vi "FMA1600A General Setup.vi"(5 "Gas Type":T5, 6 "Baud Rate":T2(ring)=enum."19200", 7 "Unit ID":string, 8 "error in (no error)":errorcluster, 9 "Select Gas?":bool=TRUE, 10 "Set STP Register":bool, 11 "VISA Refnum in":refnum<visa-resource-name>) -> (0 "error out":errorcluster, 1 "Data Frame Format":T1, 2 "Measurement Units":T3, 3 "VISA Refnum out":refnum<visa-resource-name>)   [LabVIEW 2019]
uses:
  Type Definitions/FMA1600A Gas Type.ctl
  Type Definitions/FMA1600A Units String.ctl
  Alicat Gas Meter Driver/Sub-VIs/Units of Measure.ctl
  Alicat Gas Meter Driver/Sub-VIs/Data Frame.ctl
  Type Definitions/FMA1600A Commands.ctl
  <vilib>/Utility/error.llb/whitespace.ctl
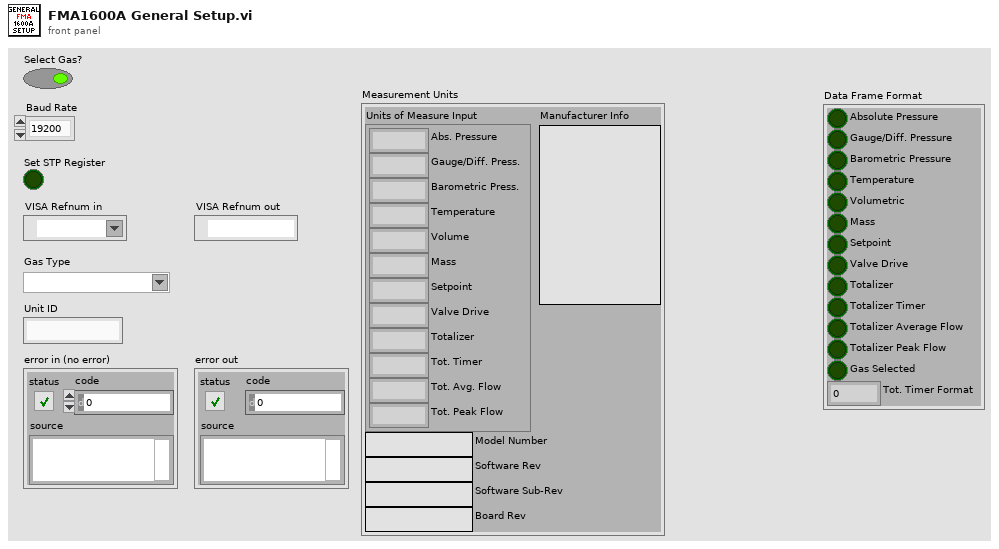
[diagram p1: front panel]
types:
  T1 = typedef "Data Frame.ctl" = cluster{"Absolute Pressure":bool, "Gauge/Diff. Pressure":bool, "Barometric Pressure":bool, "Temperature":bool, "Volumetric":bool, "Mass":bool, "Setpoint":bool, "Valve Drive":bool, "Totalizer":bool, "Totalizer Timer":bool, "Totalizer Average Flow":bool, "Totalizer Peak Flow":bool, "Gas Selected":bool, "Tot. Timer Format":u16}
  T2 = enum8{"2400", "9600", "19200", "38400", "57600", "115200", "Unknown"}
  T3 = typedef "FMA1600A Units String.ctl" = cluster{"Software Rev":string, "Model Number":string, "Manufacturer Info":string, "Software Sub-Rev":string, "Board Rev":string, "Units of Measure Input":T4}
  T4 = typedef "Units of Measure.ctl" = cluster{"Abs. Pressure":string, "Gauge/Diff. Press.":string, "Barometric Press.":string, "Temperature":string, "Volume":string, "Mass":string, "Setpoint":string, "Valve Drive":string, "Totalizer":string, "Tot. Timer":string, "Tot. Avg. Flow":string, "Tot. Peak Flow":string}
  T5 = typedef "FMA1600A Gas Type.ctl" = string
  T6 = cluster{"Valve Drive":bool, "Totalizer":bool, "Totalizer Timer":bool, "Totalizer Peak Flow":bool, "Show Abs., Gauge\nand Baro. pressures":bool}
  T7 = cluster{"Pressure(s)":bool, "Temperature":bool, "Volumetric":bool, "Mass":bool, "Totalizer Average Flow":bool, "Gas Selected":bool}
  T8 = typedef "whitespace.ctl" = u16
  T9 = typedef "FMA1600A Commands.ctl" = string
  T10 = cluster{"Unit ID":string, "Baud Rate":enum8{"2400", "9600", "19200", "38400", "57600", "115200", "Unknown"}, "VISA Sesssion In":refnum<visa-resource-name>}
  T11 = cluster{"Abs. Pressure":string, "Gauge/Diff. Press.":string, "Barometric Press.":string, "Temperature":string, "Volume":string, "Mass":string, "Setpoint":string, "Valve Drive":string, "Totalizer":string, "Tot. Timer":string, "Tot. Avg. Flow":string, "Tot. Peak Flow":string}
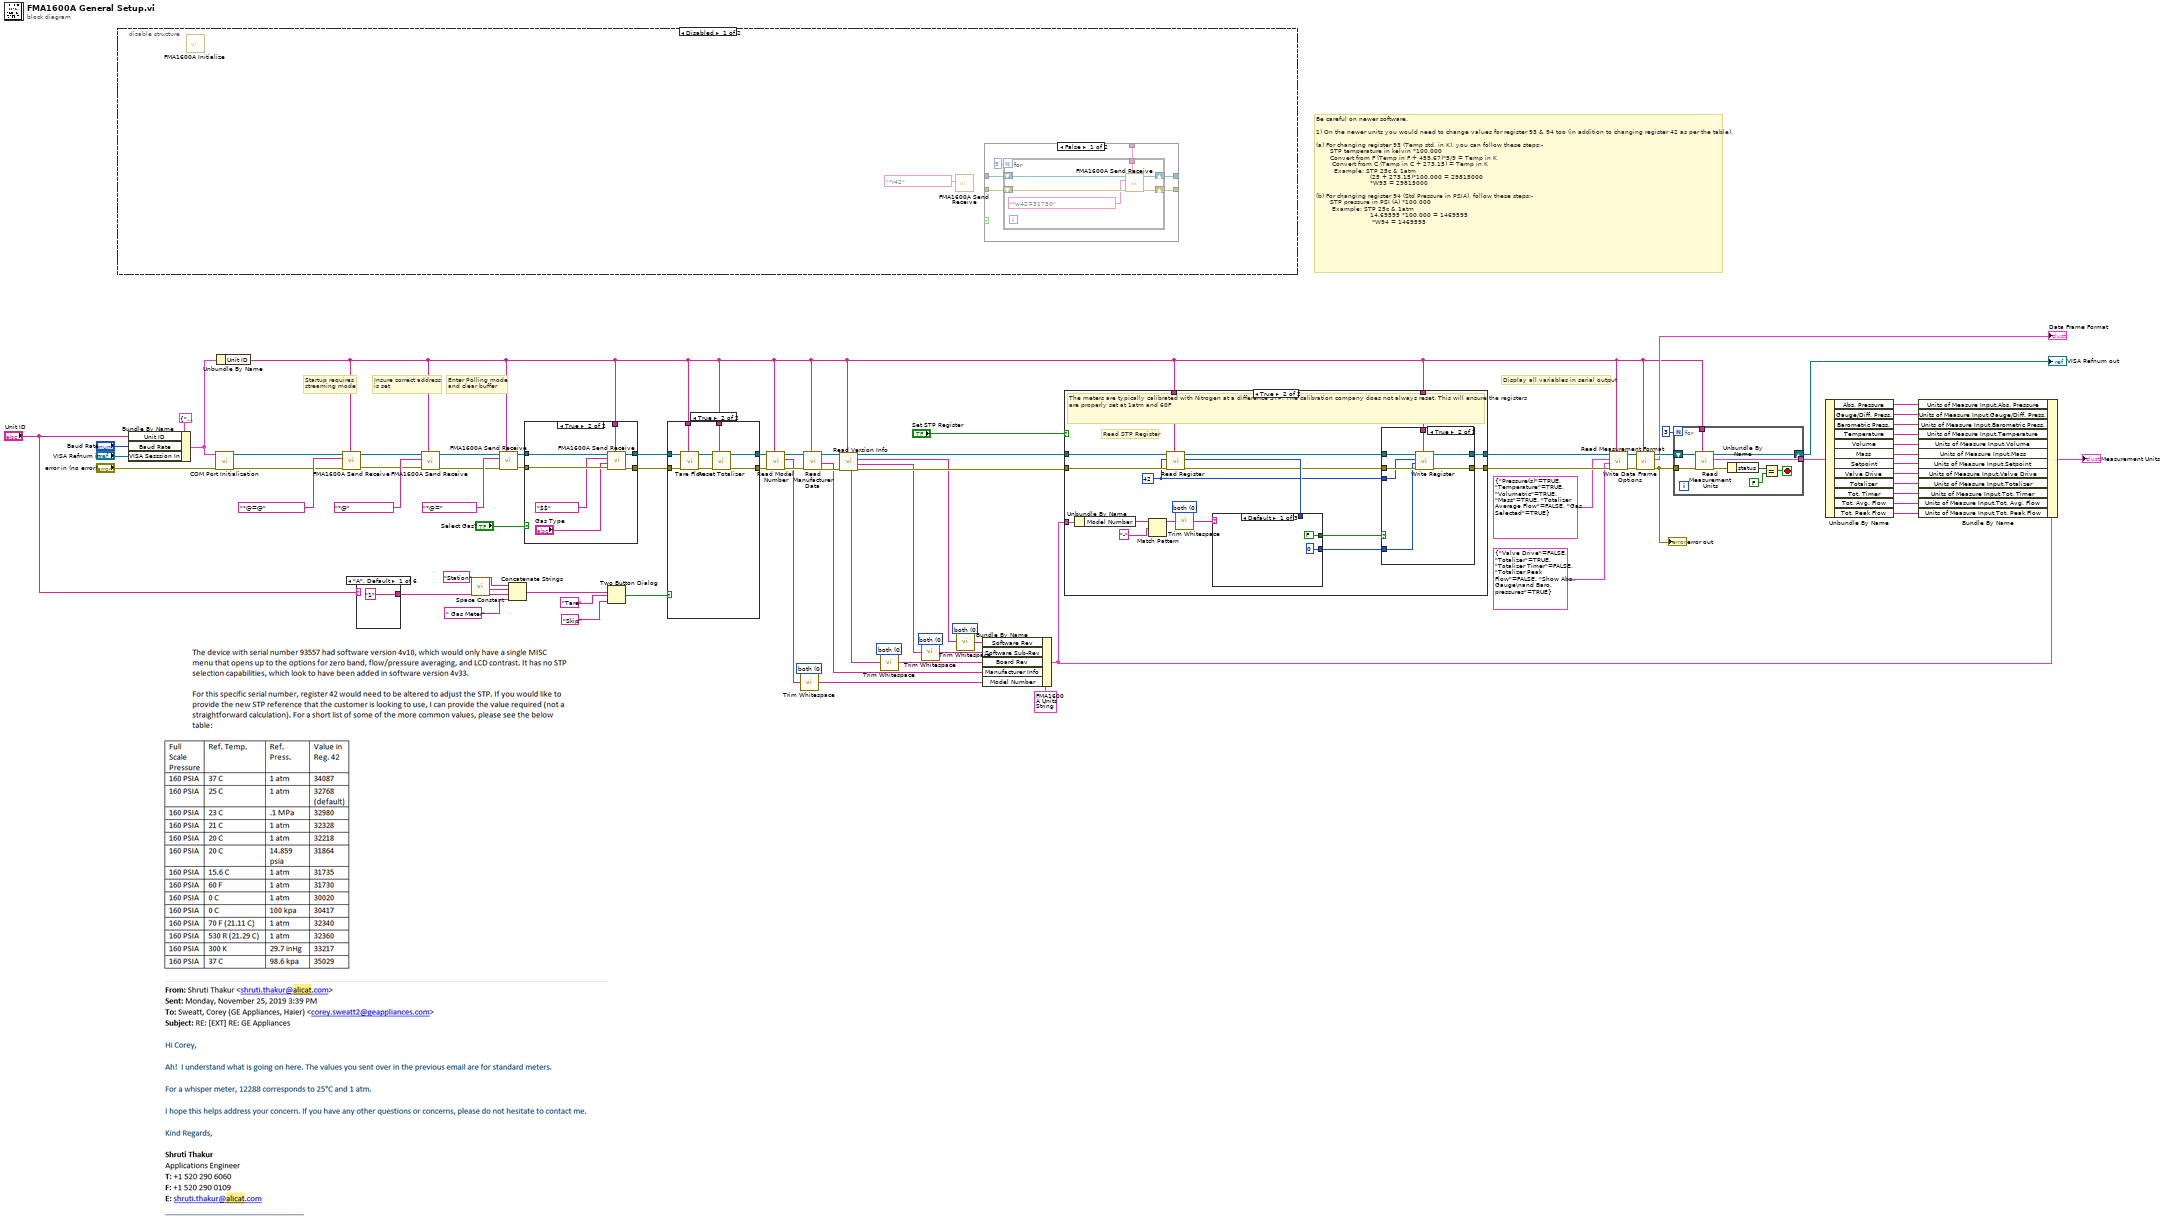
[diagram p0: block diagram]
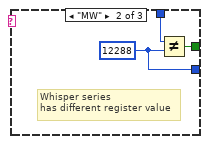
[diagram p7: hidden frame]
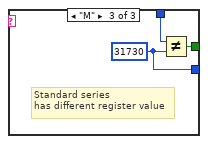
[diagram p8: hidden frame]
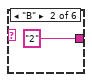
[diagram p9: hidden frame]
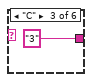
[diagram p10: hidden frame]
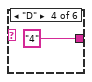
[diagram p11: hidden frame]
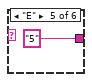
[diagram p12: hidden frame]
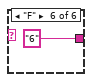
[diagram p13: hidden frame]
diagram:
  w13 = T8 0 items=["both", "start of string", "end of string"] ("location (both)")
  w14 = T8 0 items=["both", "start of string", "end of string"] ("location (both)")
  w17 = T8 0 items=["both", "start of string", "end of string"] ("location (both)")
  w18 = T8 0 items=["both", "start of string", "end of string"] ("location (both)")
  # "Display all variables in serial output"
  # "Enter Polling mode\nand clear buffer"
  # "Startup requires \nstreaming mode"
  # "Insure correct address\nis set"
  # "Be careful on newer software.\n\n1) On the newer units you would need to change values for register 93 & 94 too (in addition to changing register 42 as per the table). \n\n(a) For changing register 93 (Temp std. in K), you can follow these steps:-\n       STP temperature in kelvin *100,000\n       Convert from F (Temp in F + 459.67)*5/9 = Temp in K\n        Convert from C (Temp in C + 273.15) = Temp in K\n         Example: STP 25c & 1atm\n                           (25 + 273.15)*100,000 = 29815000\n                           *W93 = 29815000\n\n(b) For changing register 94 (Std Pressure in PSIA), follow these steps:-\n       STP pressure in PSI (A) *100,000\n        Example: STP 25c & 1atm\n                           14.69595 *100,000 = 1469595\n                            *W94 = 1469595"
  n1 = disable-structure shown="Disabled" {
    frame Disabled {
      n2 = call "FMA1600A Initialize.vi"() -> ()  [unwired: 10 in, 2 out]
      n3 = call "FMA1600A Send Receive.vi"("FMA1600A Commands"=T9 "*r42") -> ()  [unwired: 8 in, 3 out]
      n4 = case shown="False" {
        selector: _ -> [_ _]
        tunnel: [w85 w92] -> _
        tunnel: [w84 w93] -> _
        tunnel: _ -> [w83 _]
        tunnel: _ -> [w81 w92]
        tunnel: _ -> [w80 w93]
        frame False {
          n5 = for {
            N: 5 -> [_]
            tunnel: w83 -> [w87]
            shift-right: [w90] -> w84
            shift-left: w80 -> [w89]
            shift-right: [w91] -> w85
            shift-left: w81 -> [w88]
            n6 = call "FMA1600A Send Receive.vi"("Unit ID"=w87, "error in (no error)"=w89, "FMA1600A Commands"=T9 "*w42=31730", "VISA Refnum in"=w88) -> ("error out"=w90:errorcluster, "VISA Refnum out"=w91:refnum<visa-resource-name>)  [unwired: 5 in, 1 out]
          }
        }
        frame True {
        }
      }
    }
    frame Enabled {
    }
  }
  n7 = Bundle By Name(cluster=T10 {"Unit ID"="A", "Baud Rate"=enum."19200", "VISA Sesssion In"="COM1"} ("Communication Settings"), "Unit ID"="Unit ID", "Baud Rate"="Baud Rate", "VISA Sesssion In"="VISA Refnum in") -> (w62:T10)
  n8 = call "COM Port Initialization.vi"("error in (no error)"="error in (no error)", "Communication Settings"=w62) -> ("error out"=w59:errorcluster, "VISA Session Out"=w58:refnum<visa-resource-name>)  [unwired: 8 in]
  n9 = Unbundle By Name(w62) -> ("Unit ID"=w4:string)
  n10 = call "FMA1600A Send Receive.vi"("Unit ID"=w4, "error in (no error)"=w59, "FMA1600A Commands"=T9 "*@=@", "VISA Refnum in"=w58) -> ("error out"=w57:errorcluster, "VISA Refnum out"=w56:refnum<visa-resource-name>)  [unwired: 5 in, 1 out]
  n11 = case shown="\"A\", Default" "Unit ID" {
    tunnel: ["1" ("message") "2" ("message") "3" ("message") "4" ("message") "5" ("message") "6" ("message")] -> w76
    frame "A", Default {
    }
    frame "B" {
    }
    frame "C" {
    }
    frame "D" {
    }
    frame "E" {
    }
    frame "F" {
    }
  }
  n12 = call "FMA1600A Send Receive.vi"("Unit ID"=w4, "error in (no error)"=w57, "FMA1600A Commands"=T9 "*@", "VISA Refnum in"=w56) -> ("error out"=w51:errorcluster, "VISA Refnum out"=w52:refnum<visa-resource-name>)  [unwired: 5 in, 1 out]
  n13 = call <vilib>:"Space Constant.vi"() -> ("String"=w70:string)
  n14 = call "FMA1600A Send Receive.vi"("Unit ID"=w4, "error in (no error)"=w51, "FMA1600A Commands"=T9 "*@=", "VISA Refnum in"=w52) -> ("error out"=w55:errorcluster, "VISA Refnum out"=w54:refnum<visa-resource-name>)  [unwired: 5 in, 1 out]
  n15 = Concatenate Strings("Station" ("message"), w70, w76, " Gas Meter" ("string")) -> (w73:string)
  n16 = case shown="True" "Select Gas?" {
    tunnel: w55 -> [w101 w108]
    tunnel: w54 -> [w100 w107]
    tunnel: [w100 w104] -> w50
    tunnel: [w101 w103] -> w49
    tunnel: w4 -> [_ w102]
    frame False {
    }
    frame True {
      n17 = call "FMA1600A Send Receive.vi"("Unit ID"=w102, "error in (no error)"=w108, "Gas Type"="Gas Type", "FMA1600A Commands"=T9 "$$", "VISA Refnum in"=w107) -> ("error out"=w103:errorcluster, "VISA Refnum out"=w104:refnum<visa-resource-name>)  [unwired: 4 in, 1 out]
    }
  }
  n18 = Two Button Dialog(message=w73, 1:"Skip" ("F button name (\"Cancel\")"), 2:"Tare" ("T button name (\"OK\")")) -> (T button?=w78:bool)
  n19 = case shown="True" w78 {
    tunnel: [w109 w111] -> w33
    tunnel: [w110 w112] -> w34
    tunnel: w49 -> [w110 w117]
    tunnel: w50 -> [w109 w116]
    tunnel: w4 -> [_ w118]
    tunnel: w4 -> [_ w113]
    frame False {
    }
    frame True {
      n20 = call "Tare Flow.vi"("Unit ID (A)"=w118, "error in"=w117, "VISA Session In"=w116) -> ("error out"=w115:errorcluster, "VISA Session Out"=w114:refnum<visa-resource-name>)  [unwired: 7 in]
      n21 = call "Reset Totalizer.vi"("Unit ID (A)"=w113, "error in"=w115, "VISA Session In"=w114) -> ("error out"=w112:errorcluster, "VISA Session Out"=w111:refnum<visa-resource-name>)  [unwired: 6 in, 1 out]
    }
  }
  n22 = call "Read Model Number.vi"("Unit ID (A)"=w4, "error in"=w34, "VISA Session In"=w33) -> ("error out"=w32:errorcluster, "Model Number"=w20:string, "VISA Session Out"=w31:refnum<visa-resource-name>)  [unwired: 6 in]
  n23 = call <vilib>:"Trim Whitespace.vi"("string"=w20, "location (both)"=w18) -> ("trimmed string"=w19:string)
  n24 = call "Read Manufacturer Data.vi"("Unit ID (A)"=w4, "error in"=w32, "VISA Session In"=w31) -> ("error out"=w29:errorcluster, "Manufacturer Info"=w25:string, "VISA Session Out"=w30:refnum<visa-resource-name>)  [unwired: 6 in]
  n25 = call "Read Version Info.vi"("Unit ID (A)"=w4, "error in"=w29, "VISA Session In"=w30) -> ("error out"=w28:errorcluster, "Software Sub-Rev"=w12:string, "Software Rev"=w16:string, "VISA Session Out"=w27:refnum<visa-resource-name>, "Board Rev"=w10:string)  [unwired: 4 in]
  n26 = call <vilib>:"Trim Whitespace.vi"("string"=w10, "location (both)"=w14) -> ("trimmed string"=w9:string)
  n27 = call <vilib>:"Trim Whitespace.vi"("string"=w12, "location (both)"=w13) -> ("trimmed string"=w11:string)
  n28 = call <vilib>:"Trim Whitespace.vi"("string"=w16, "location (both)"=w17) -> ("trimmed string"=w15:string)
  n29 = Bundle By Name(cluster=T3 {"Software Rev"="", "Model Number"="", "Manufacturer Info"="", "Software Sub-Rev"="", "Board Rev"="", "Units of Measure Input"={"Abs. Pressure"="", "Gauge/Diff. Press."="", "Barometric Press."="", "Temperature"="", "Volume"="", "Mass"="", "Setpoint"="", "Valve Drive"="", "Totalizer"="", "Tot. Timer"="", "Tot. Avg. Flow"="", "Tot. Peak Flow"=""}} ("Measurement Units"), "Software Rev"=w15, "Software Sub-Rev"=w11, "Board Rev"=w9, "Manufacturer Info"=w25, "Model Number"=w19) -> (w24:T3)
  n30 = case shown="True" "Set STP Register" {
    tunnel: [w119 w125] -> w6
    tunnel: [w120 w128] -> w8
    tunnel: w28 -> [w120 w137]
    tunnel: w27 -> [w119 w138]
    tunnel: w4 -> [_ w121]
    tunnel: w4 -> [_ w127]
    tunnel: w24 -> [_ w136]
    frame False {
    }
    frame True {
      w132 = T8 0 items=["both", "start of string", "end of string"] ("location (both)")
      w124 = u16 42 ("Register address")
      # "Read STP Register"
      # "The meters are typically calibrated with Nitrogen at a difference STP. The calibration company does not always reset. This will ensure the registers are properly set at 1atm and 60F"
      n31 = Unbundle By Name(w136) -> ("Model Number"=w135:string)
      n32 = Match Pattern(string=w135, regular expression="-" ("search string")) -> (before substring=w133:string)  [unwired: 1 in, 3 out]
      n33 = call "Read Register.vi"("Unit ID (A)"=w121, "error in"=w137, "Register address"=w124, "VISA Session In"=w138) -> ("error out"=w129:errorcluster, "Register Value (I32)"=w130:i32, "VISA Session Out"=w126:refnum<visa-resource-name>)  [unwired: 5 in]
      n34 = call <vilib>:"Trim Whitespace.vi"("string"=w133, "location (both)"=w132) -> ("trimmed string"=w131:string)
      n35 = case shown="Default" w131 {
        tunnel: w130 -> [_ w152 w155]
        tunnel: [FALSE w151 w154] -> w122
        tunnel: [0 ("y") w150 w153] -> w123
        frame Default {
        }
        frame "MW" {
          w150 = 12288 ("y")
          # "Whisper series\nhas different register value"
          n36 = Not Equal?(x=w152, y=w150) -> (x != y?=w151:bool)
        }
        frame "M" {
          w153 = 31730 ("y")
          # "Standard series\nhas different register value"
          n37 = Not Equal?(x=w155, y=w153) -> (x != y?=w154:bool)
        }
      }
      n38 = case shown="True" w122 {
        tunnel: w129 -> [w140 w147]
        tunnel: [w140 w146] -> w128
        tunnel: w127 -> [_ w145]
        tunnel: w126 -> [w139 w144]
        tunnel: [w139 w143] -> w125
        tunnel: w124 -> [_ w142]
        tunnel: w123 -> [_ w141]
        frame False {
        }
        frame True {
          n39 = call "Write Register.vi"("Unit ID (A)"=w145, "error in"=w147, "Register Value"=w141, "Register address"=w142, "VISA Session In"=w144) -> ("error out"=w146:errorcluster, "VISA Session Out"=w143:refnum<visa-resource-name>)  [unwired: 4 in, 1 out]
        }
      }
    }
  }
  n40 = call "Write Data Frame Options.vi"("Unit ID (A)"=w4, "error in"=w8, "Enables: Data frame only"=T6 {"Valve Drive"=FALSE, "Totalizer"=TRUE, "Totalizer Timer"=FALSE, "Totalizer Peak Flow"=FALSE, "Show Abs., Gauge\nand Baro. pressures"=TRUE}, "Enables: \nData frame and Display"=T7 {"Pressure(s)"=TRUE, "Temperature"=TRUE, "Volumetric"=TRUE, "Mass"=TRUE, "Totalizer Average Flow"=FALSE, "Gas Selected"=TRUE} ("Enables: \nData frame and Display"), "VISA Session In"=w6) -> ("error out"=w7:errorcluster, "VISA Session Out"=w5:refnum<visa-resource-name>)  [unwired: 5 in]
  n41 = call "Read Measurement Format.vi"("Unit ID (A)"=w4, "error in"=w7, "VISA Session In"=w5) -> ("error out"=w21:errorcluster, "Data Frame Format"=→"Data Frame Format":T1, "VISA Session Out"=w23:refnum<visa-resource-name>)  [unwired: 6 in]
  "error out" <- w21
  n42 = for {
    N: 3 -> [_]
    tunnel: w4 -> [w158]
    tunnel: [w160] -> w48
    shift-right: [w161] -> w69
    shift-left: w23 -> [w162]
    tunnel: w21 -> [w159]
    stop <- w163 stop-if-true
    n43 = call "Read Measurement Units.vi"("Unit ID (A)"=w158, "error in"=w159, "VISA Session In"=w162) -> ("error out"=w164:errorcluster, "Measurement Units"=w160:T11, "VISA Session Out"=w161:refnum<visa-resource-name>)  [unwired: 5 in, 1 out]
    n44 = Unbundle By Name(w164) -> ("status"=w157:bool)
    n45 = Equal?(x=w157, y=FALSE ("x")) -> (x = y?=w163:bool)
  }
  "VISA Refnum out" <- w69
  n46 = Unbundle By Name(w48) -> ("Abs. Pressure"=w46:string, "Gauge/Diff. Press."=w45:string, "Barometric Press."=w44:string, "Temperature"=w43:string, "Volume"=w42:string, "Mass"=w41:string, "Setpoint"=w40:string, "Valve Drive"=w39:string, "Totalizer"=w38:string, "Tot. Timer"=w37:string, "Tot. Avg. Flow"=w36:string, "Tot. Peak Flow"=w35:string)
  n47 = Bundle By Name(cluster=w24, "Units of Measure Input.Abs. Pressure"=w46, "Units of Measure Input.Gauge/Diff. Press."=w45, "Units of Measure Input.Barometric Press."=w44, "Units of Measure Input.Temperature"=w43, "Units of Measure Input.Volume"=w42, "Units of Measure Input.Mass"=w41, "Units of Measure Input.Setpoint"=w40, "Units of Measure Input.Valve Drive"=w39, "Units of Measure Input.Totalizer"=w38, "Units of Measure Input.Tot. Timer"=w37, "Units of Measure Input.Tot. Avg. Flow"=w36, "Units of Measure Input.Tot. Peak Flow"=w35) -> (→"Measurement Units":T3)
